vi "Pre Launch Init.vi"(11 "UserInterface in":refnum<class "UserInterface.lvclass">) -> (0 "error out":errorcluster, 3 "UserInterface out":refnum<class "UserInterface.lvclass">)   [LabVIEW 2016, in "UserInterface.lvlib" / "UserInterface.lvclass"]
doc: "(<B>Filename</B>: Actor Framework.lvlib:Actor.lvclass:Pre Launch Init.vi)\n\nDefines behavior that occurs after the Launch Nested Actor method is invoked but before the actor's Actor Core method begins running.\n\nBy default, this method does nothing. A descendant class may override it to define behavior."
uses:
  UserInterface.lvclass
  UserInterface.lvclass/UserInterface.ctl
  <vilib>/ActorFramework/Actor/Actor.lvclass
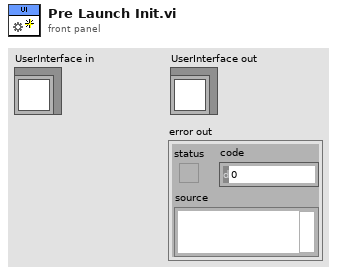
[diagram p1: front panel]
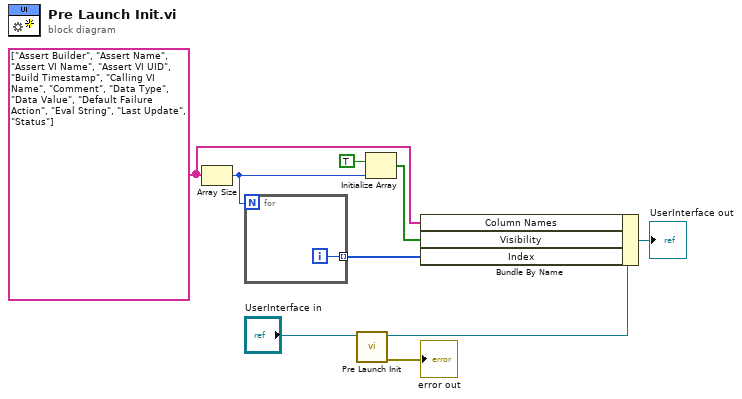
[diagram p0: block diagram]
diagram:
  w5 = string[] ["Assert Builder", "Assert Name", "Assert VI Name", "Assert VI UID", "Build Timestamp", "Calling VI Name", "Comment", "Data Type", "Data Value", "Default Failure Action", "Eval String", "Last Update", "Status"] ("sorted array")
  n1 = Array Size(array=w5) -> (size(s)=w2:i32)
  n2 = for {
    N: w2 -> [_]
    tunnel: [w10] -> w1 mode=indexing
    i -> [w10]
  }
  n3 = call-parent "Pre Launch Init.vi"("Actor in"="UserInterface in") -> ("error out"=→"error out":errorcluster, "Actor out"=w8:refnum<class "UserInterface.lvclass">)  [unwired: 9 in]
  n4 = Initialize Array(TRUE, w2) -> (w3:bool[])
  n5 = Bundle By Name(cluster=w8, "Column Names"=w5, "Visibility"=w3, "Index"=w1) -> (→"UserInterface out":refnum<class "UserInterface.lvclass">)
